vi "collapse_dist_mid_collapse_dist_welding_20KHZ.vi"() -> ()   [LabVIEW 2017]
uses:
  Generic_Common/WeldAutomation/Global_Variable_Status_Indicator.vi
panel:
  out "Weld Status":bool
  out "Status indicator main":string
  out "Pre part contanct in inch":dbl
  out "Pre Part Contanct distance in mm pre":dbl
  out "Absolute distance in inch":dbl
  out "Absolute distance in mm":dbl
  out "#Iterations:":dbl format="%-#1.6g"
  out "Welding Progress":u8(slide) scale=0.0..100.0
  out "Test Result":picture
  out "Performance Graph":cluster{dbl, u32}[](graph)
  # "Instructions:\n1. Make sure Ethernet cable from SC board connected to Laptop, \n2. Type netstat in command pompt to cross verify, SC port connection is established \n3. Then run the VI, press palm button first time button for actuator setup FPC will be perfomed\n4. Again press palm button to perform welding, second time onward welding will be perfomed\n5, To edit local_config.ini file to change the recipe parameters."
  # "Test execution sequence : \n1. Read SC, PC_AC parameters from INI file\n2. Send command to BL\n    a. MessageID_SC + Length (SC parameters) + SC parameters\n      b. MessageID_PC_AC  + Length (PC_AC parameters) + PC_AC parameters\n3. Receive response from BL after sending recipe parameters\n      c. ResponseID + Message \n4. Press palm button using USB6008 device\n5. Report Generation and Log generation"
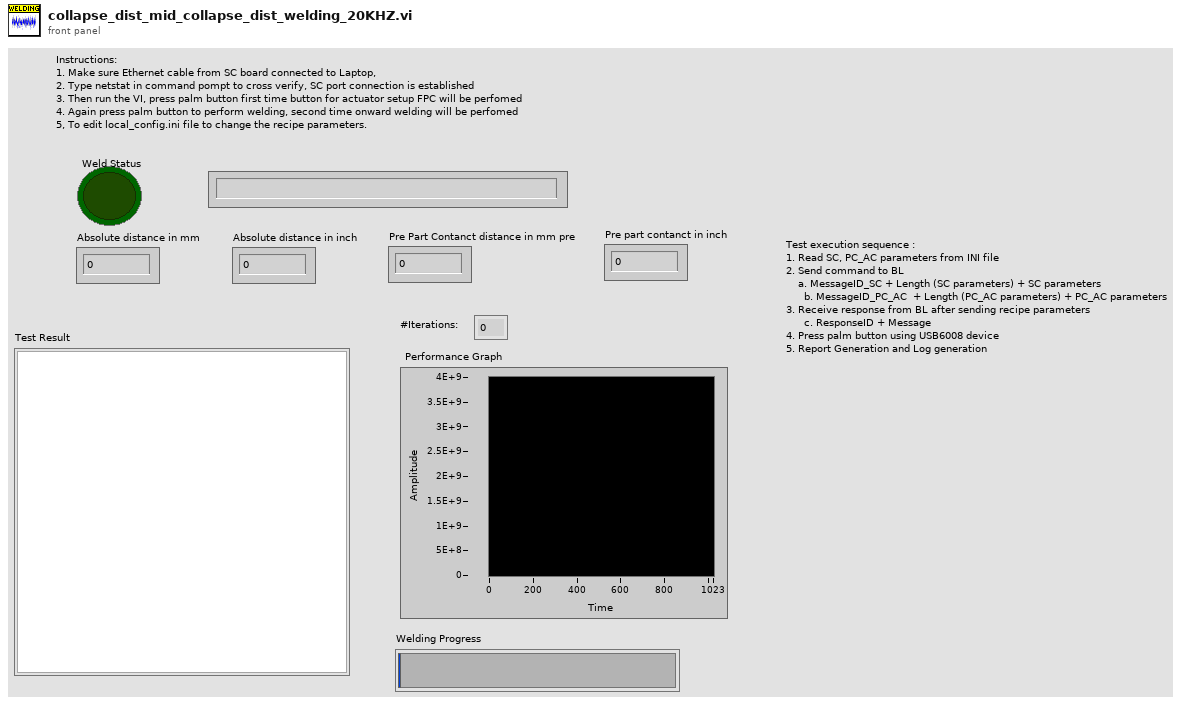
[diagram p1: front panel]
types:
  T1 = enum16{"open", "replace", "create", "open or create", "replace or create", "replace or create with confirmation"}
  T2 = cluster{"[0]":string, "[1]":string, "[2]":string, "[3]":string, "[4]":string, "[5]":string, "[6]":string, "[7]":string, "[8]":string}
  T3 = cluster{"Socket_IP_Address":string, "Socket_Port_Number":u16, "Global_ReportPath":path}
  T4 = typedef "imagedata.ctl" = cluster{"image type":i32, "image depth":i32, "image":u8[], "mask":u8[], "colors":u32[], "Rectangle":cluster{"left":i16, "top":i16, "right":i16, "bottom":i16}}
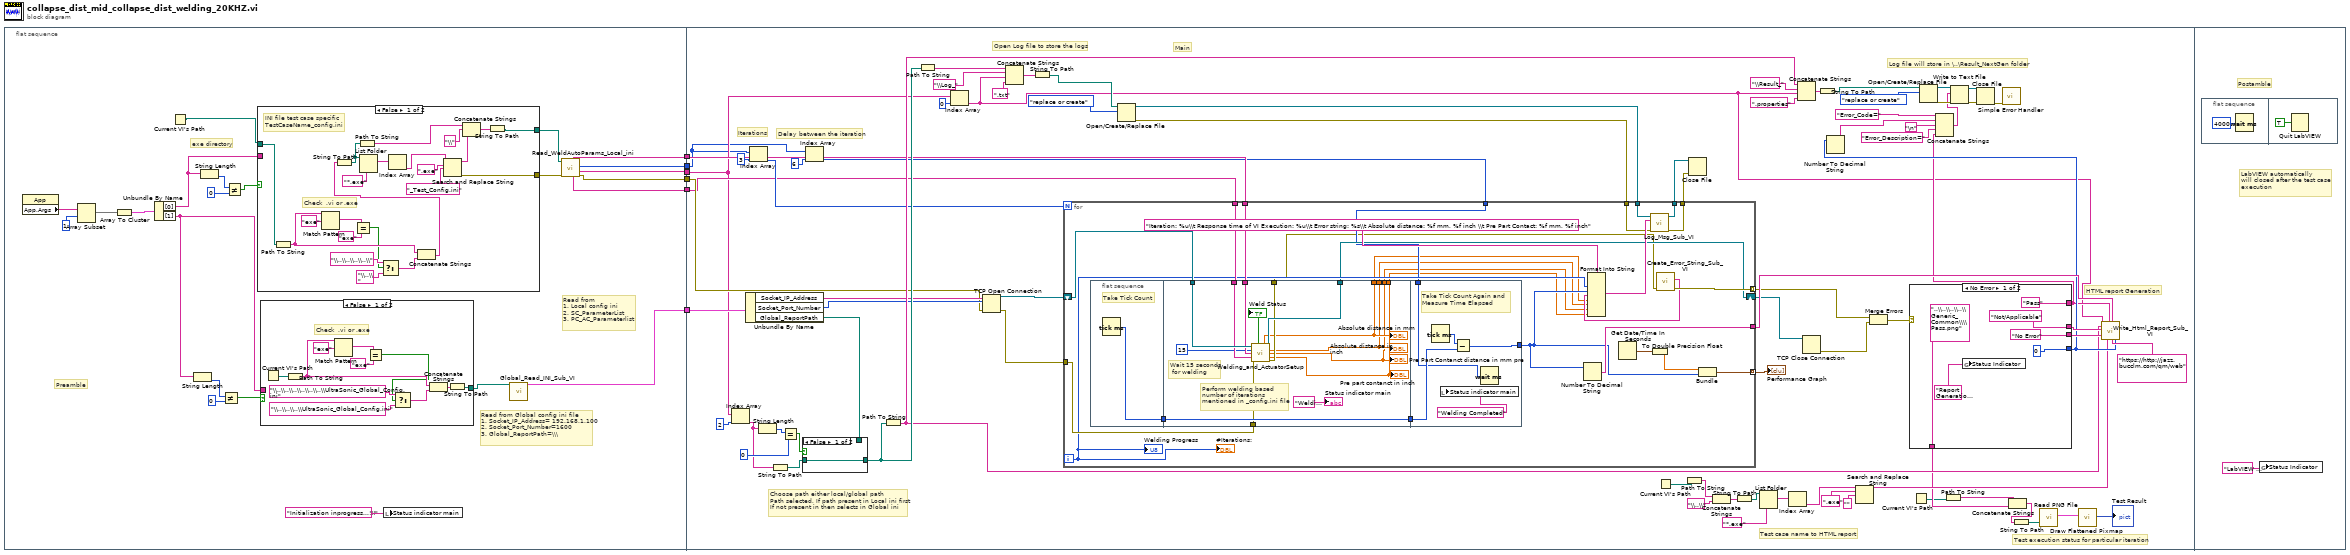
[diagram p0: block diagram]
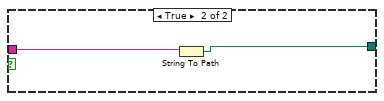
[diagram p2: hidden frame]
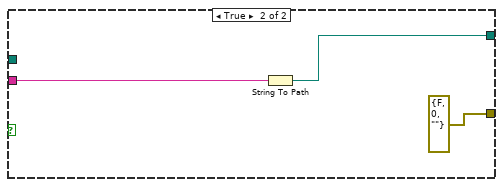
[diagram p3: hidden frame]
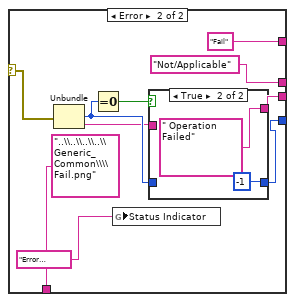
[diagram p5: hidden frame]
diagram:
  n1 = flat-sequence {
    tunnel: [w13] -> w6
    tunnel: [w15] -> w5
    tunnel: [w12] -> w4
    tunnel: [w11] -> w3
    tunnel: [w10] -> w2
    tunnel: [w9] -> w1
    tunnel: w6 -> [w88]
    tunnel: w5 -> [w93]
    tunnel: w4 -> [w73]
    tunnel: w3 -> [w77]
    tunnel: w2 -> [w76]
    tunnel: w1 -> [w75]
    frame #0 {
      # "exe directory"
      # "Read from Global config ini file\n1. Socket_IP_Address= 192.168.1.100\n2. Socket_Port_Number=1600\n3. Global_ReportPath=\\\\\\"
      # "Read from\n1. Local config ini\n2. SC_ParameterList\n3. PC_AC_Parameterlist"
      # "Preamble"
      n2 = property class="App"() -> ("App.Args"=w17:string[])  [unwired: 2 in, 2 out]
      n3 = Array Subset "Array Subset"(array=w17, index=1) -> (w18:string[])  [unwired: 1 in]
      n4 = Array To Cluster(array=w18) -> (cluster=w19:T2)
      n5 = Unbundle By Name "Unbundle By Name"(w19) -> ("[0]"=w23:string, "[1]"=w26:string)
      n6 = Current VI's Path() -> (path=w7:path)
      n7 = String Length(string=w26) -> (length=w27:i32)
      n8 = String Length(string=w23) -> (length=w20:i32)
      n9 = Not Equal?(x=w27, y=0) -> (x != y?=w25:bool)
      n10 = Not Equal?(x=w20, y=0) -> (x != y?=w22:bool)
      n11 = case shown="False" w22 {
        tunnel: w23 -> [_ w67]
        tunnel: [w56 w66] -> w28
        tunnel: [w55 errorcluster {"status"=FALSE, "code"=0, "source"=""} ("error out")] -> w14
        tunnel: w7 -> [w44 _]
        frame False {
          # "Check  .vi or .exe"
          # "INI file test case specific\nTestCaseName_config.ini"
          n12 = Path To String(path=w44) -> (string=w49:string)
          n13 = Match Pattern(string=w49, regular expression="exe") -> (match substring=w48:string)  [unwired: 1 in, 3 out]
          n14 = Equal?(x=w48, y="exe") -> (x = y?=w46:bool)
          n15 = Select(t="\\..\\..\\..\\..\\" ("string"), s=w46, f="\\..\\" ("string")) -> (s? t:f=w50:string)
          n16 = Concatenate Strings(w49, w50) -> (w43:string)
          n17 = String To Path(string=w43) -> (path=w54:path)
          n18 = Path To String(path=w54) -> (string=w53:string)
          n19 = List Folder(path=w54, pattern="*.exe") -> (filenames=w58:string[])  [unwired: 2 in, 3 out]
          n20 = Index Array(array=w58) -> (element=w57:string)  [unwired: 1 in]
          n21 = Search and Replace String(input string=w57, search string=".exe", replace string="_Test_Config.ini" ("replace string (\"\")")) -> (result string=w62:string, error out=w55:errorcluster)  [unwired: 5 in, 2 out]
          n22 = Concatenate Strings(w53, "\\" ("string"), w62) -> (w60:string)
          n23 = String To Path(string=w60) -> (path=w56:path)
        }
        frame True {
          n24 = String To Path(string=w67) -> (path=w66:path)
        }
      }
      n25 = case shown="False" w25 {
        tunnel: [w39 w42] -> w29
        tunnel: w26 -> [_ w41]
        frame False {
          # "Check  .vi or .exe"
          n26 = Current VI's Path() -> (path=w31:path)
          n27 = Path To String(path=w31) -> (string=w35:string)
          n28 = Match Pattern(string=w35, regular expression="exe") -> (match substring=w34:string)  [unwired: 1 in, 3 out]
          n29 = Equal?(x=w34, y="exe") -> (x = y?=w32:bool)
          n30 = Select(t="\\..\\..\\..\\..\\..\\..\\UltraSonic_Global_Config.ini" ("string"), s=w32, f="\\..\\..\\..\\UltraSonic_Global_Config.ini" ("string")) -> (s? t:f=w36:string)
          n31 = Concatenate Strings(w35, w36) -> (w40:string)
          n32 = String To Path(string=w40) -> (path=w39:path)
        }
        frame True {
          n33 = String To Path(string=w41) -> (path=w42:path)
        }
      }
      n34 = local write "Status indicator main"("Initialization inprogress...!!!" ("Current status")) -> ()
      n35 = call "Global_Read_INI_Sub_VI.vi"("Config File Path"=w29) -> ("output cluster"=w15:T3)  [unwired: 14 in]
      n36 = call "Read_WeldAutoParams_Local_ini.vi"("TestCaseName_Config.ini File Path (Test case level)"=w28, "error in"=w14) -> ("SC Parameters to BL (HEX format)"=w11:string, "PC_AC Parameters to BL (HEX format)"=w10:string, "[Initialization]"=w12:i32[], "[framework_settings]"=w9:string[], "error out"=w13:errorcluster)  [unwired: 4 in]
    }
    frame #1 {
      # "Delay between the iteration"
      # "Open Log file to store the logs"
      # "HTML report Generation"
      # "Log file will store in \\..\\Result_NextGen folder"
      # "Test execution status for particular iteration"
      # "Test case name to HTML report"
      # "Iterations"
      # "Choose path either local/global path\nPath selected, If path present in Local ini first\nIf not present in then selects in Global ini"
      # "Main"
      n37 = Index Array(array=w75, index=2) -> (element=w82:string)
      n38 = Unbundle By Name(w93) -> ("Socket_IP_Address"=w90:string, "Socket_Port_Number"=w89:u16, "Global_ReportPath"=w92:path)
      n39 = Index Array(array=w73, index=3) -> (element=w78:i32)
      n40 = String Length(string=w82) -> (length=w136:i32)
      n41 = String To Path(string=w82) -> (path=w81:path)
      n42 = Equal?(x=w136, y=0) -> (x = y?=w134:bool)
      n43 = case shown="False" w134 {
        tunnel: w92 -> [_ w148]
        tunnel: [w147 w148] -> w133
        tunnel: w81 -> [w147 _]
        frame False {
        }
        frame True {
        }
      }
      n44 = Index Array(array=w73, index=6) -> (element=w72:i32)
      n45 = Path To String(path=w133) -> (string=w110:string)
      n46 = Path To String(path=w133) -> (string=w138:string)
      n47 = Index Array(array=w75, index=0) -> (element=w68:string)
      n48 = TCP Open Connection(address=w90, remote port or service name=w89, error in (no error)=w88) -> (connection ID=w85:refnum<k5>, error out=w87:errorcluster)  [unwired: 2 in]
      n49 = Concatenate Strings(w138, "\\Log_" ("string"), w68, ".txt" ("string")) -> (w141:string)
      n50 = String To Path(string=w141) -> (path=w140:path)
      n51 = Open/Create/Replace File(file path (use dialog)=w140, operation (0:open)=T1."replace or create") -> (refnum out=w111:refnum<file>, error out=w114:errorcluster)  [unwired: 1 in, 4 out]
      n52 = for {
        N: w78 -> [_]
        tunnel: [w174] -> w144
        tunnel: w111 -> [w168]
        tunnel: [w167] -> w113
        tunnel: [w165] -> w112
        tunnel: [w170] -> w142 mode=indexing
        tunnel: w114 -> [w166]
        tunnel: [w163] -> w109 mode=indexing
        tunnel: w87 -> [w161]
        shift-right: [w156] -> w86
        shift-left: w85 -> [w160]
        tunnel: w77 -> [w159]
        tunnel: w76 -> [w158]
        tunnel: w72 -> [w155]
        i -> [w157]
        n53 = flat-sequence {
          tunnel: [w176] -> w175
          tunnel: [w190] -> w154
          tunnel: w175 -> [w190]
          tunnel: w161 -> [w186]
          tunnel: w160 -> [w189]
          tunnel: w159 -> [w187]
          tunnel: w158 -> [w188]
          tunnel: [w185] -> w156
          tunnel: [w184] -> w153
          tunnel: [w182] -> w152
          tunnel: [w181] -> w151
          tunnel: [w180] -> w150
          tunnel: [w179] -> w149
          tunnel: w154 -> [w195]
          tunnel: [w193] -> w164
          tunnel: w155 -> [w192]
          frame #0 {
            # "Take Tick Count"
            n54 = Tick Count (ms)() -> (millisecond timer value=w176:u32)
          }
          frame #1 {
            # "Wait 15 seconds\n for welding"
            # "Perform welding based \nnumber of iterations\nmentioned in _config.ini file"
            n55 = call "Welding_and_ActuatorSetup.vi"("TCP connection IN"=w189, "Number of second to wait"=15, "SC_7"=w187, "ACPC_8"=w188, "Error In"=w186) -> ("Weld Status"=→"Weld Status":bool, "Absolute distance in mm"=w182:dbl, "TCP connection OUT"=w185:refnum<k5>, "Absolute distance in inch"=w181:dbl, "Prepart contact in mm"=w180:dbl, "Prepart contact in inch"=w179:dbl, "Error Out"=w184:errorcluster)  [unwired: 2 in, 2 out]
            "Absolute distance in mm" <- w182
            "Absolute distance in inch" <- w181
            "Pre Part Contanct distance in mm pre" <- w180
            "Pre part contanct in inch" <- w179
            "Status indicator main" <- "Welding Inprogress...!!!"
          }
          frame #2 {
            # "Take Tick Count Again and Measure Time Elapsed"
            n56 = Tick Count (ms)() -> (millisecond timer value=w194:u32)
            n57 = local write "Status indicator main"("Welding Completed" ("Current status")) -> ()
            n58 = Subtract(x=w194, y=w195) -> (x-y=w193:u32)
            n59 = Wait (ms)(milliseconds to wait=w192) -> ()  [unwired: 1 out]
          }
        }
        n60 = Number To Decimal String(number=w164) -> (decimal integer string=w174:string)  [unwired: 1 in]
        n61 = Get Date/Time In Seconds() -> (seconds since 1Jan1904=w171:timestamp)
        n62 = To Double Precision Float(number=w171) -> (double precision float=w172:dbl)
        n63 = call "Create_Error_String_Sub_VI.vi"("error in"=w153) -> ("error out"=w163:errorcluster, "Error String"=w162:string)  [unwired: 9 in]
        n64 = Format Into String(format string="Iteration: %u\\t Response time of VI Execution: %u\\t Error string: %s\\t Absolute distance: %f mm, %f inch \\t Pre Part Contact: %f mm, %f inch", w157, w164, w162, w152, w151, w150, w149) -> (resulting string=w169:string)  [unwired: 2 in, 1 out]
        n65 = call "Log_Msg_Sub_VI.vi"("error in (no error)"=w166, "String"=w169, "Byte Stream File in"=w168) -> ("error out"=w165:errorcluster, "Byte Stream File out"=w167:refnum<file>)  [unwired: 7 in]
        n66 = Bundle "Bundle"(w172, w164) -> (w170:cluster{dbl, u32})  [unwired: 1 in]
        "Welding Progress" <- w157
        "#Iterations:" <- w157
      }
      "Performance Graph" <- w142
      n67 = Current VI's Path() -> (path=w69:path)
      n68 = Path To String(path=w69) -> (string=w106:string)
      n69 = Close File(refnum=w113, error in=w112) -> ()  [unwired: 2 out]
      n70 = Concatenate Strings(w106, "\\..\\" ("string")) -> (w104:string)
      n71 = String To Path(string=w104) -> (path=w108:path)
      n72 = List Folder(path=w108, pattern="*.exe") -> (filenames=w103:string[])  [unwired: 2 in, 3 out]
      n73 = Index Array(array=w103) -> (element=w99:string)  [unwired: 1 in]
      n74 = Concatenate Strings(w110, "\\Result_" ("string"), w68, ".properties" ("string")) -> (w131:string)
      n75 = TCP Close Connection(connection ID=w86) -> (error out=w84:errorcluster)  [unwired: 2 in, 1 out]
      n76 = String To Path(string=w131) -> (path=w123:path)
      n77 = Search and Replace String(input string=w99, search string=".exe", replace string="" ("replace string (\"\")")) -> (result string=w102:string)  [unwired: 5 in, 3 out]
      n78 = Merge Errors "Merge Errors"(w109, w84) -> (w91:errorcluster)
      n79 = case shown="No Error" w91 {
        selector: w91 -> [_ w202]
        tunnel: ["Pass" "Fail"] -> w115
        tunnel: [0 ("code") w206] -> w119
        tunnel: ["No Error" ("source") w207] -> w146
        tunnel: ["Not/Applicable" "Not/Applicable"] -> w145
        tunnel: ["..\\..\\..\\..\\Generic_Common\\\\Pass.png" ("string") "..\\..\\..\\..\\Generic_Common\\\\Fail.png" ("string")] -> w94
        frame No Error {
          n80 = global write "Global_Variable_Status_Indicator.vi" "Status Indicator"("Report Generation inprogress...!!!" ("Current status")) -> ()
        }
        frame Error {
          n81 = Unbundle(w202) -> ("code"=w208:i32, "source"=w204:string)  [unwired: 1 out]
          n82 = Equal To 0?(x=w208) -> (x = 0?=w205:bool)
          n83 = global write "Global_Variable_Status_Indicator.vi" "Status Indicator"("Error occurred, Report Generation inprogress...!!!" ("Current status")) -> ()
          n84 = case shown="True" w205 {
            tunnel: [w213 -1 ("code")] -> w206
            tunnel: [w212 " Operation Failed" ("source")] -> w207
            tunnel: w208 -> [w213 _]
            tunnel: w204 -> [w212 _]
            frame False {
            }
            frame True {
            }
          }
        }
      }
      n85 = Number To Decimal String(number=w119) -> (decimal integer string=w118:string)  [unwired: 1 in]
      n86 = Current VI's Path() -> (path=w71:path)
      n87 = Open/Create/Replace File(file path (use dialog)=w123, operation (0:open)=T1."replace or create") -> (refnum out=w122:refnum<file>, error out=w127:errorcluster)  [unwired: 4 in, 1 out]
      n88 = Concatenate Strings("Error_Code=" ("string"), w118, "\n", "Error_Description=" ("string"), w115) -> (w121:string)
      n89 = Path To String(path=w71) -> (string=w70:string)
      n90 = Write to Text File(file (use dialog)=w122, text=w121, error in=w127) -> (refnum out=w126:refnum<file>, error out=w125:errorcluster)  [unwired: 1 in, 1 out]
      n91 = Close File(refnum=w126, error in=w125) -> (error out=w124:errorcluster)  [unwired: 1 out]
      n92 = call <vilib>:"Simple Error Handler.vi"("error in (no error)"=w124) -> ()  [unwired: 4 in, 5 out]
      n93 = Concatenate Strings(w70, w94) -> (w95:string)
      n94 = String To Path(string=w95) -> (path=w98:path)
      n95 = call <vilib>:"Read PNG File.vi"("path to PNG file"=w98) -> ("image data"=w96:T4)  [unwired: 8 in, 2 out]
      n96 = call <vilib>:"Draw Flattened Pixmap.vi"("image data"=w96) -> ("new picture"=→"Test Result":picture)  [unwired: 8 in]
      n97 = call "Write_Html_Report_Sub_VI.vi"("ReprtPath"=w110, "Remarks"=w145, "Error Description"=w146, "Timestamp"=w68, "TestCase"=w102, "Verdict"=w115, "Time taken to execute  test in msec"=w144, "JazzDashboardLink"="https://http://jazz.bucclm.com/qm/web" ("TestSuite"), "Error Code"=w119) -> ()  [unwired: 11 in]
    }
    frame #2 {
      # "LabVIEW automatically\nwill closed after the test case \nexecution"
      # "Postamble"
      n98 = flat-sequence {
        frame #0 {
          n99 = Wait (ms)(milliseconds to wait=u32 4000) -> ()  [unwired: 1 out]
        }
        frame #1 {
          n100 = Quit LabVIEW(quit? (T)=TRUE) -> ()
        }
      }
      n101 = global write "Global_Variable_Status_Indicator.vi" "Status Indicator"("LabVIEW VI Closing off...!!!" ("Current status")) -> ()
    }
  }
